vi "alter database password.vi"(8 "错误输入（无错误）":errorcluster, 9 "NewPWd":string, 10 "OpenPwd":string, 11 "路径":path) -> (0 "错误输出":errorcluster)   [LabVIEW 2016, in "Access Lib.lvlib"]
uses:
  Access Lib.lvlib
  <vilib>/addons/database/Connection.llb/DB Tools Open Connec (String).vi
  <vilib>/addons/database/Connection.llb/Conn Execute.vi
  <vilib>/addons/database/Recordset.llb/Rec Destroy - Connection.vi
  <vilib>/addons/database/NI_Database_API.lvlib
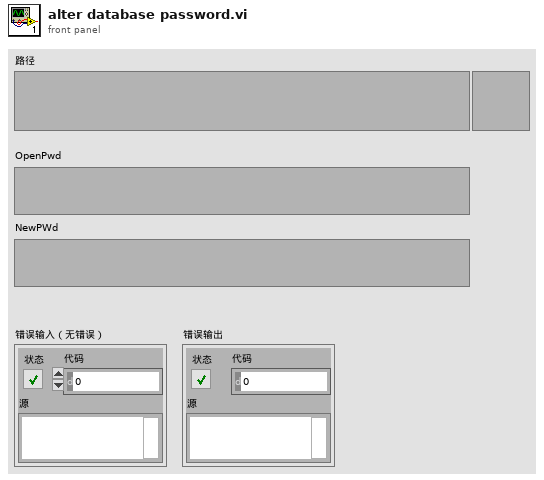
[diagram p1: front panel]
types:
  T1 = typedef "NI_Database_API.lvlib/Conn ObjectReference.ctl" = refnum<k1>
  T2 = typedef "NI_Database_API.lvlib/Rec ObjectReference.ctl" = refnum<k1>
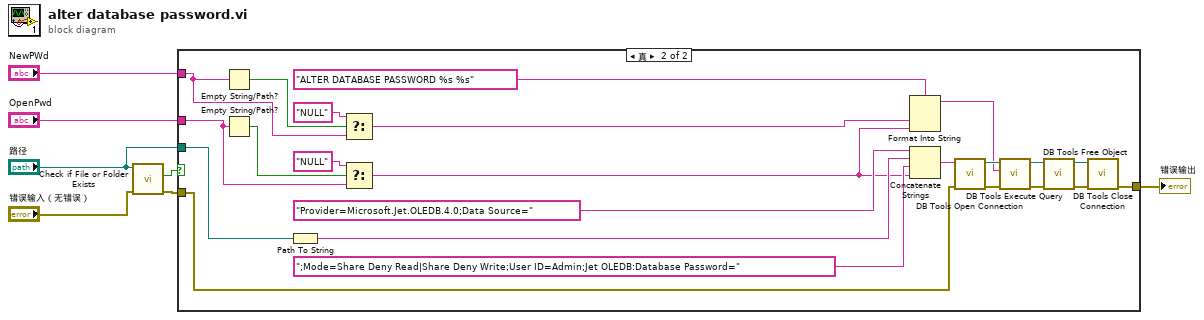
[diagram p0: block diagram]
diagram:
  n1 = call <vilib>:"Check if File or Folder Exists.vi"("error in (no error)"="错误输入（无错误）", "path"="路径") -> ("error out"=w3:errorcluster, "file or folder exists?"=w5:bool)  [unwired: 7 in, 1 out]
  n2 = case shown="真" w5 {
    tunnel: "OpenPwd" -> [_ w11]
    tunnel: "路径" -> [_ w28]
    tunnel: w3 -> [w8 w19]
    tunnel: [w8 w20] -> w2
    tunnel: "NewPWd" -> [_ w14]
    frame False {
    }
    frame True {
      n3 = Empty String/Path?(string/path=w14) -> (empty?=w16:bool)
      n4 = Empty String/Path?(string/path=w11) -> (empty?=w12:bool)
      n5 = Path To String(path=w28) -> (string=w31:string)
      n6 = Select(t="NULL", s=w16, f=w14) -> (s? t:f=w10:string)
      n7 = Select(t="NULL", s=w12, f=w11) -> (s? t:f=w9:string)
      n8 = Format Into String(format string="ALTER DATABASE PASSWORD %s %s" ("格式字符串"), w10, w9) -> (resulting string=w17:string)  [unwired: 2 in, 1 out]
      n9 = Concatenate Strings("Provider=Microsoft.Jet.OLEDB.4.0;Data Source=" ("ConnectString"), w31, ";Mode=Share Deny Read|Share Deny Write;User ID=Admin;Jet OLEDB:Database Password=" ("字符串"), w9) -> (w27:string)
      n10 = call-poly <vilib>:"DB Tools Open Connection.vi"("error in (no error)"=w19, "connection information"=w27) -> ("error out"=w25:errorcluster, "connection reference"=w26:T1)  [unwired: 6 in]
      n11 = call-poly <vilib>:"DB Tools Execute Query.vi"("error in (no error)"=w25, "SQL query"=w17, "connection reference"=w26) -> ("error out"=w23:errorcluster, "recordset reference"=w24:T2)  [unwired: 5 in]
      n12 = call-poly <vilib>:"DB Tools Free Object.vi"("error in (no error)"=w23, "recordset reference"=w24) -> ("error out"=w21:errorcluster, "connection reference"=w22:T1)  [unwired: 8 in]
      n13 = call <vilib>:"DB Tools Close Connection.vi"("error in (no error)"=w21, "connection reference"=w22) -> ("error out"=w20:errorcluster)  [unwired: 5 in]
    }
  }
  "错误输出" <- w2
